vi "VernierTemp.vi"() -> ()   [LabVIEW 2019]
uses:
  <userlib>/MicroPython/VIs/uPythonX/uPythonX.xctl
panel:
  in  "Combined":T1(xcontrol)={"Port"="HighPeaksPYBD - ASRL114::INSTR", "All Code"="import micropython\nfrom bluetooth import BLE, UUID, FLAG_NOTIFY, FLAG_READ, FLAG_WRITE, FLAG_NOTIFY\nfrom micropython import const\nimport time\nimport struct\n\nmicropython.alloc_emergency_exception_buf(100)\n\nimport gc,utime\nimport pyb, micropython\nimport LPF2Class\n\n# Name, Format [# datasets, type, figures, decimals], raw [min,max], Percent, SI, Symbol,functionMap, view\nmode0 = ['LPF2-DETECT',[1,LPF2Class.DATA8,3,0],[0,10],[0,100],[0,10],'',[LPF2Class.ABSOLUTE,0],True]\nmode1 = ['LPF2-COUNT',[1,LPF2Class.DATA8,4,0],[0,100],[0,100],[0,100],'CNT',[LPF2Class.ABSOLUTE,0],True]\nmode2 = ['LPF2-CAL',[3,LPF2Class.DATA16,3,0],[0,1023],[0,100],[0,1023],'RAW',[LPF2Class.ABSOLUTE,0],False]\nmodes = [mode0,mode1,mode2]\n\nred_led=pyb.LED(1)\ngreen_led = pyb.LED(2)\nred_led.on()\n\nlpf2 = LPF2Class.LPF2(1, 'Y1', 'Y2', modes, 35, timer = 4, freq = 5)    # PyBoard\nlpf2.initialize()\n\nwhile True:\n     if not lpf2.connected:\n          lpf2.sendTimer.callback(None)\n          red_led.on()\n          utime.sleep_ms(200)\n          lpf2.initialize()\n     else:\n          red_led.off()\n          lpf2.current_mode = 0\n          lpf2.load_payload_char(4)\n          break\n\n#For debug, specify sensor to be found here:\nGDX_SENSOR_ORDER_CODE = \"GDX-TMP\" #Found on product label\nGDX_SENSOR_SN_LAST3 = \"4S7\"      #Last 3 digits of serial number found on product label\n\n# Bluetooth IRQ handler states. Commented out Subscriber conditions since this is for a central\n#_IRQ_CENTRAL_CONNECT                 = const(1 << 0)\n#_IRQ_CENTRAL_DISCONNECT              = const(1 << 1)\n#_IRQ_GATTS_WRITE                     = const(1 << 2)\n#_IRQ_GATTS_READ_REQUEST              = const(1 << 3)\n_IRQ_SCAN_RESULT                     = const(1 << 4)\n_IRQ_SCAN_COMPLETE                   = const(1 << 5)\n_IRQ_PERIPHERAL_CONNECT              = const(1 << 6)\n_IRQ_PERIPHERAL_DISCONNECT           = const(1 << 7)\n_IRQ_GATTC_SERVICE_RESULT            = const(1 << 8)\n_IRQ_GATTC_CHARACTERISTIC_RESULT     = const(1 << 9)\n_IRQ_GATTC_DESCRIPTOR_RESULT         = const(1 << 10)\n_IRQ_GATTC_READ_RESULT               = const(1 << 11)\n_IRQ_GATTC_WRITE_STATUS              = const(1 << 12)\n_IRQ_GATTC_NOTIFY                    = const(1 << 13)\n_IRQ_GATTC_INDICATE                  = const(1 << 14)\n\n#Go Direct specific UUIDs for D2PIO (our protocol) communication.\nSERVICE_UUID                        = \"d91714ef-28b9-4f91-ba16-f0d9a604f112\"\nCMD_CHARACTERISTIC_UUID             = \"f4bf14a6-c7d5-4b6d-8aa8-df1a7c83adcb\"\nRESPONSE_CHARACTERISTIC_UUID        = \"b41e6675-a329-40e0-aa01-44d2f444babe\"\n\n#Go Direct command and expected responses\nINIT                                = b'\\x58\\x19\\xfe\\x3f\\x1a\\xa5\\x4a\\x06\\x49\\x07\\x48\\x08\\x47\\x09\\x46\\x0a\\x45\\x0b\\x44\\x0c\\x43\\x0d\\x42\\x0e\\x41'\nINIT_RESPONSE                       = b'\\xb8\\x1a\\x00\\xe0\\x1a\\xfe\\x55\\xaa\\x56\\xa9\\x57\\xa8\\x58\\xa7\\x59\\xa6\\x5a\\xa5\\x5b\\xa4\\x5c\\xa3\\x5d\\xa2\\x5e\\xa1'\nGET_STATUS_CMD                      = b'\\x58\\x05\\xfd\\x6a\\x10'\n#GET_STATUS_RESPONSE                 = b'\\x98\\x12\\x01\\x0d\\x10\\xfd\\x00\\x00\\x04\\x01\\x00\\x00\\x04\\x01\\x00\\x00\\x4b\\x00' Example only. State/Sensor dependent\nAVAILABLE_CHANNELS_CMD              = b'\\x58\\x05\\xfc\\xaa\\x51'\n#AVAILABLE_CHANNELS_RESP             = b'\\x98\\x0a\\x01\\xf4\\x51\\xfe\\x02\\x00\\x00\\x00' Example only. State/Sensor dependent\n#sample period of 0.1 sec  = 01 86 a0\n#smaple period of 1.0 sec  = 0f 42 40\nSET_MEASUREMENT_PERIOD_CMD          = b'\\x58\\x0f\\xfb\\xa3\\x1b\\xff\\x00\\x40\\x42\\x0f\\x00\\x00\\x00\\x00\\x00'\n#SET_MEASUREMENT_PERIOD_RESP         = b'\\x98\\x10\\x03\\xe7\\x1b\\xfb \\xff\\x00\\xa0\\x86\\x01\\x00\\x00\\x00\\x00\\x00' Example only. State/Sensor dependent\nSTART_MEASUREMENTS_CMD              = b'\\x58\\x13\\xfa\\x7f\\x18\\xff\\x01\\x02\\x00\\x00\\x00\\x00\\x00\\x00\\x00\\x00\\x00\\x00\\x00'\n#START_MEASUREMENTS_CMD              = b'\\x58\\x13\\xfa\\x7f\\x18\\xff\\x00\\x02\\x00\\x00\\x00\\x00\\x00\\x00\\x00\\x00\\x00\\x00\\x00'\n#START_MEASUREMENTS_RESP             = b'\\x98\\x07\\x04\\xb5\\x18\\xfa\\x00' Example only. State/Sensor dependent\nSTOP_MEASUREMENTS_CMD               = b'\\x58\\x0b\\xf9\\x70\\x19\\xff\\x00\\xff\\xff\\xff\\xff'\nSTOP_MEASUREMENTS_RESP              = b'\\x98\\x07\\x05\\xb6\\x19\\xf9\\x00'\n\n\nglobal scanning_flag\nscanning_flag = False\n\nclass BLEPeripheral:\n  def __init__(self):\n    self._addr_type = None\n    self._addr = bytearray(5)\n    self._conn_handle = None\n    self._connect_status = False\n    self._rssi = None\n    self._name = None\n    #characteristic info from querry\n    self._cmdhandle = 20\n    self._resphandle = 22\n    self._command = bytearray()\n    self._response = bytearray()\n    #D2PIO Protocol\n    self._rolling_counter = None\n\n  def connected(self):\n   pass\n\n\ndef adv_decode(adv_type, data):\n    i = 0\n    while i + 1 < len(data):\n        if data[i + 1] == adv_type:\n            return data[i + 2:i + data[i] + 1]\n        i += 1 + data[i]\n    return None\n\ndef adv_decode_name(data):\n    n = adv_decode(0x09, data)\n    if n:\n        return n.decode('utf-8')\n    return data\n\ndef bt_irq(event, data):\n  global scanning_flag\n  if event == _IRQ_SCAN_RESULT:\n    # A single scan result.\n    addr_type, addr, connectable, rssi, adv_data = data\n    if adv_decode_name(adv_data).startswith(GDX_SENSOR_ORDER_CODE) and connectable:\n        if adv_decode_name(adv_data).endswith(GDX_SENSOR_SN_LAST3):\n            print(addr_type, addr, connectable, rssi, adv_decode_name(adv_data))\n            bledevice._addr[:] = addr\n            bledevice._addr_type = addr_type\n            bledevice._rssi = rssi\n        pass\n  elif event == _IRQ_SCAN_COMPLETE:\n    # Scan duration finished or manually stopped.\n    #print('scan complete')\n    scanning_flag = False\n    pass\n  elif event == _IRQ_PERIPHERAL_CONNECT:\n    # A successful gap_connect().\n    conn_handle, addr_type, addr = data\n    bledevice._conn_handle = conn_handle\n    print(\"Connected to \" + str(conn_handle) + str(addr_type))\n    scanning_flag = False\n  elif event == _IRQ_PERIPHERAL_DISCONNECT:\n    # A successful gap_connect().\n    conn_handle, addr_type, addr = data\n    print(\"Disconnected\")\n    scanning_flag = False\n  elif event == _IRQ_GATTC_SERVICE_RESULT:\n    # Called for each service found by gattc_discover_services().\n    conn_handle, start_handle, end_handle, uuid = data\n    print(\"Service\", conn_handle, start_handle, end_handle, uuid)\n    scanning_flag = False\n  elif event == _IRQ_GATTC_CHARACTERISTIC_RESULT:\n    # Called for each characteristic found by gattc_discover_services().\n    conn_handle, def_handle, value_handle, properties, uuid = data\n    print(\"Characteristic\", conn_handle, def_handle, value_handle, properties, uuid)\n    scanning_flag = False\n  elif event == _IRQ_GATTC_DESCRIPTOR_RESULT:\n    # Called for each characteristic found by gattc_discover_services().\n    conn_handle, dsc_handle, uuid = data\n    print(\"Descriptor\", conn_handle, dsc_handle, uuid)\n    scanning_flag = False\n  elif event == _IRQ_GATTC_READ_RESULT:\n    # A gattc_read() has completed.\n    conn_handle, value_handle, char_data = data\n    bledevice._response[:] = char_data            \n    print(conn_handle, value_handle, char_data)\n    scanning_flag = False\n  elif event == _IRQ_GATTC_WRITE_STATUS:\n    # A gattc_write() has completed.\n    conn_handle, value_handle, status = data\n    print(\"Data write\" , conn_handle, value_handle, status)\n    scanning_flag = False\n  elif event == _IRQ_GATTC_NOTIFY:\n    # A peripheral has sent a notify request.\n    conn_handle, value_handle, notify_data = data\n #   print(\"Notify\", value_handle, notify_data)\n #   if conn_handle == bledevice._conn_handle and value_handle == bledevice._resphandle:\n    bledevice._response[:] = notify_data\n    scanning_flag = False\n  else :\n    print(\"IRQ Number\", event)\n\n\ndef GDX_calculate_checksum(buff):\n    length = int(buff[1])\n    checksum = -1 * int(buff[3])\n\n    for i in range(0,length):\n        checksum += int(buff[i])\n        checksum = checksum & 0xFF\n\n        if checksum < 0 or checksum > 255:\n            return 0\n\n    return checksum\n\ndef GDX_SendInit(PassedBLEDevice):\n    # Reset the rolling packet counter\n    PassedBLEDevice._rolling_counter = 0xFF\n    PassedBLEDevice._command = INIT\n    # Populate the packet header bytes\n    workinglist = list(PassedBLEDevice._command)\n    workinglist[1] = len(PassedBLEDevice._command)\n    workinglist[2] = PassedBLEDevice._rolling_counter\n    PassedBLEDevice._rolling_counter = PassedBLEDevice._rolling_counter -1\n    workinglist[3] = 0 \n    workinglist[3] = GDX_calculate_checksum(workinglist)\n    PassedBLEDevice._command = bytearray(workinglist)\n    scanning_flag = True\n    bt.gattc_write(PassedBLEDevice._conn_handle, PassedBLEDevice._cmdhandle, PassedBLEDevice._command,True)\n    return\n\ndef GDX_GetStatus(PassedBLEDevice):\n    PassedBLEDevice._command = GET_STATUS_CMD\n    # Populate the packet header bytes\n    workinglist = list(PassedBLEDevice._command)\n    workinglist[1] = len(PassedBLEDevice._command)\n    workinglist[2] = PassedBLEDevice._rolling_counter\n    PassedBLEDevice._rolling_counter = PassedBLEDevice._rolling_counter -1\n    workinglist[3] = 0 \n    workinglist[3] = GDX_calculate_checksum(workinglist)\n    PassedBLEDevice._command = bytearray(workinglist)\n    print(\"GetStatus CMD\", PassedBLEDevice._command)\n    bt.gattc_write(PassedBLEDevice._conn_handle, PassedBLEDevice._cmdhandle, PassedBLEDevice._command,True)\n    return\n\ndef GDX_AvalCh(PassedBLEDevice):\n    PassedBLEDevice._command = AVAILABLE_CHANNELS_CMD\n    # Populate the packet header bytes\n    workinglist = list(PassedBLEDevice._command)\n    workinglist[1] = len(PassedBLEDevice._command)\n    workinglist[2] = PassedBLEDevice._rolling_counter\n    PassedBLEDevice._rolling_counter = PassedBLEDevice._rolling_counter -1\n    workinglist[3] = 0 \n    workinglist[3] = GDX_calculate_checksum(workinglist)\n    PassedBLEDevice._command = bytearray(workinglist)\n    print(\"Available Channels CMD\", PassedBLEDevice._command)\n    bt.gattc_write(PassedBLEDevice._conn_handle, PassedBLEDevice._cmdhandle, PassedBLEDevice._command,True)\n    return\n\ndef GDX_SetPeriod(PassedBLEDevice):\n    bt2 = BLE()\n    PassedBLEDevice._command = SET_MEASUREMENT_PERIOD_CMD\n    workinglist = list(PassedBLEDevice._command)\n    workinglist[1] = len(PassedBLEDevice._command)\n    workinglist[2] = PassedBLEDevice._rolling_counter\n    PassedBLEDevice._rolling_counter = PassedBLEDevice._rolling_counter -1\n    workinglist[3] = 0 \n    workinglist[3] = GDX_calculate_checksum(workinglist)\n    PassedBLEDevice._command = bytearray(workinglist)\n    print(\"Set Period\", PassedBLEDevice._command, PassedBLEDevice._conn_handle, PassedBLEDevice._cmdhandle)\n    bt2.gattc_write(PassedBLEDevice._conn_handle, PassedBLEDevice._cmdhandle, PassedBLEDevice._command,True)\n    return\n\ndef GDX_StartMeasurement(PassedBLEDevice):\n    bt2 = BLE()\n    PassedBLEDevice._command = START_MEASUREMENTS_CMD\n    workinglist = list(PassedBLEDevice._command)\n    workinglist[1] = len(PassedBLEDevice._command)\n    workinglist[2] = PassedBLEDevice._rolling_counter\n    PassedBLEDevice._rolling_counter = PassedBLEDevice._rolling_counter -1\n    workinglist[3] = 0 \n    workinglist[3] = GDX_calculate_checksum(workinglist)\n    PassedBLEDevice._command = bytearray(workinglist)\n    print(\"Start Measurements\", PassedBLEDevice._command, PassedBLEDevice._conn_handle, PassedBLEDevice._cmdhandle)\n    bt2.gattc_write(PassedBLEDevice._conn_handle, PassedBLEDevice._cmdhandle, PassedBLEDevice._command,True)\n    return\n\ndef GDX_StopMeasurement(PassedBLEDevice):\n    PassedBLEDevice._command = STOP_MEASUREMENTS_CMD\n    # Populate the packet header bytes\n    workinglist = list(PassedBLEDevice._command)\n    workinglist[1] = len(PassedBLEDevice._command)\n    workinglist[2] = PassedBLEDevice._rolling_counter\n    PassedBLEDevice._rolling_counter = PassedBLEDevice._rolling_counter -1\n    workinglist[3] = 0 \n    workinglist[3] = GDX_calculate_checksum(workinglist)\n    PassedBLEDevice._command = bytearray(workinglist)\n    bt.gattc_write(PassedBLEDevice._conn_handle, PassedBLEDevice._cmdhandle, PassedBLEDevice._command,True)\n    return\n\n'''\nTest program to take samples for 10 sec. at 1 sec. intervals\n'''\n#Scan for sensor \nbt = BLE()\nbledevice = BLEPeripheral()\nbt.irq(handler=bt_irq)\nbt.active(True)\nscanning_flag = True\nbt.gap_scan(2000, 1000, 1000)\nwhile scanning_flag:\n    pass\n\n#we have our sensor, now connect\nscanning_flag = True\nbt.gap_connect(bledevice._addr_type,bledevice._addr,)\nwhile scanning_flag:\n    pass\nprint('successful conn handle: ' + str(bledevice._conn_handle))\n\ntime.sleep_ms(500)\nbledevice._command = b'\\x01\\x00' #enable notification on characteristic\nbt.gattc_write(bledevice._conn_handle, 23, bledevice._command,False)\nwhile scanning_flag:\n    pass\nscanning_flag = True\nbt.gattc_read(bledevice._conn_handle,23)\n\nGDX_SendInit(bledevice)\n\nGDX_SetPeriod(bledevice)\n\nscanning_flag = True\nGDX_StartMeasurement(bledevice)\nwhile scanning_flag:        #wait for IRQ to clear flag\n    pass\n\nscanning_flag = True\nwhile scanning_flag:        #wait for IRQ to clear flag\n    pass\nprint(\"Start Measurements response\", bledevice._response)\n\nsamples = 0\nwhile samples < 10 :\n    scanning_flag = True\n    while scanning_flag:    #wait for IRQ to clear flag\n        pass\n    #time.sleep_ms(500)\n    samples = samples + 1\n    value = struct.unpack(\"<f\",bledevice._response[9:])[0]\n    print(\"Data sample number =\", bledevice._response[2] , struct.unpack(\"<f\",bledevice._response[9:]))\n    print(value, int(value))\nscanning_flag = True\nwhile scanning_flag:        #wait for IRQ to clear flag\n    pass\nprint(\"Measurements Stopped\")\n\n\n"}
  in  "Spike":T2(xcontrol)={"VISA Refnum in"="Spike - ASRL102::INSTR", "Python Code"="import hub,utime\n\nhub.port.B.info()\n\n# if info comes back with None - then you have to restart the pybaord\ni=0\n\nwhile True:\n     try:\n          value = hub.port.B.device.get()[0]\n          #print(value)\n          hub.display.show(str(value))\n          utime.sleep(0.1)\n     except:\n          utime.sleep(1)\n     \n"}
  in  "PYBD":T2(xcontrol)={"VISA Refnum in"="HighPeaksPYBD - ASRL114::INSTR", "Python Code"="import gc,utime\nimport pyb, micropython\nimport LPF2Class\n\nmicropython.alloc_emergency_exception_buf(200)\n\n# Name, Format [# datasets, type, figures, decimals], raw [min,max], Percent, SI, Symbol,functionMap, view\nmode0 = ['LPF2-DETECT',[1,LPF2Class.DATA8,3,0],[0,10],[0,100],[0,10],'',[LPF2Class.ABSOLUTE,0],True]\nmode1 = ['LPF2-COUNT',[1,LPF2Class.DATA8,4,0],[0,100],[0,100],[0,100],'CNT',[LPF2Class.ABSOLUTE,0],True]\nmode2 = ['LPF2-CAL',[3,LPF2Class.DATA16,3,0],[0,1023],[0,100],[0,1023],'RAW',[LPF2Class.ABSOLUTE,0],False]\nmodes = [mode0,mode1,mode2]\n\nred_led=pyb.LED(1)\ngreen_led = pyb.LED(2)\nred_led.on()\n\nlpf2 = LPF2Class.LPF2(1, 'Y1', 'Y2', modes, 35, timer = 4, freq = 5)    # PyBoard\nlpf2.initialize()\n\nvalue = 0\n\n# Loop\nwhile True:\n     if not lpf2.connected:\n          lpf2.sendTimer.callback(None)\n          red_led.on()\n          utime.sleep_ms(200)\n          lpf2.initialize()\n     else:\n          red_led.off()\n          \n          lpf2.current_mode = 0\n#          lpf2.load_payload_charArray(bytes([1,2,3,4]))\n#          lpf2.current_mode = 1\n          lpf2.load_payload_char(value)\n          \n          value = value + 1 if value <9 else 0\n          data = lpf2.readIt(timeout = 0.01)\n\n          utime.sleep_ms(90)\n"}
  in  "uPythonX":T1(xcontrol)={"Port"="HighPeaksPYBD - ASRL114::INSTR", "All Code"="import micropython\nfrom bluetooth import BLE, UUID, FLAG_NOTIFY, FLAG_READ, FLAG_WRITE, FLAG_NOTIFY\nfrom micropython import const\nimport time\nimport struct\n\nmicropython.alloc_emergency_exception_buf(100)\n\n#For debug, specify sensor to be found here:\nGDX_SENSOR_ORDER_CODE = \"GDX-TMP\" #Found on product label\nGDX_SENSOR_SN_LAST3 = \"4S7\"      #Last 3 digits of serial number found on product label\n\n# Bluetooth IRQ handler states. Commented out Subscriber conditions since this is for a central\n#_IRQ_CENTRAL_CONNECT                 = const(1 << 0)\n#_IRQ_CENTRAL_DISCONNECT              = const(1 << 1)\n#_IRQ_GATTS_WRITE                     = const(1 << 2)\n#_IRQ_GATTS_READ_REQUEST              = const(1 << 3)\n_IRQ_SCAN_RESULT                     = const(1 << 4)\n_IRQ_SCAN_COMPLETE                   = const(1 << 5)\n_IRQ_PERIPHERAL_CONNECT              = const(1 << 6)\n_IRQ_PERIPHERAL_DISCONNECT           = const(1 << 7)\n_IRQ_GATTC_SERVICE_RESULT            = const(1 << 8)\n_IRQ_GATTC_CHARACTERISTIC_RESULT     = const(1 << 9)\n_IRQ_GATTC_DESCRIPTOR_RESULT         = const(1 << 10)\n_IRQ_GATTC_READ_RESULT               = const(1 << 11)\n_IRQ_GATTC_WRITE_STATUS              = const(1 << 12)\n_IRQ_GATTC_NOTIFY                    = const(1 << 13)\n_IRQ_GATTC_INDICATE                  = const(1 << 14)\n\n#Go Direct specific UUIDs for D2PIO (our protocol) communication.\nSERVICE_UUID                        = \"d91714ef-28b9-4f91-ba16-f0d9a604f112\"\nCMD_CHARACTERISTIC_UUID             = \"f4bf14a6-c7d5-4b6d-8aa8-df1a7c83adcb\"\nRESPONSE_CHARACTERISTIC_UUID        = \"b41e6675-a329-40e0-aa01-44d2f444babe\"\n\n#Go Direct command and expected responses\nINIT                                = b'\\x58\\x19\\xfe\\x3f\\x1a\\xa5\\x4a\\x06\\x49\\x07\\x48\\x08\\x47\\x09\\x46\\x0a\\x45\\x0b\\x44\\x0c\\x43\\x0d\\x42\\x0e\\x41'\nINIT_RESPONSE                       = b'\\xb8\\x1a\\x00\\xe0\\x1a\\xfe\\x55\\xaa\\x56\\xa9\\x57\\xa8\\x58\\xa7\\x59\\xa6\\x5a\\xa5\\x5b\\xa4\\x5c\\xa3\\x5d\\xa2\\x5e\\xa1'\nGET_STATUS_CMD                      = b'\\x58\\x05\\xfd\\x6a\\x10'\n#GET_STATUS_RESPONSE                 = b'\\x98\\x12\\x01\\x0d\\x10\\xfd\\x00\\x00\\x04\\x01\\x00\\x00\\x04\\x01\\x00\\x00\\x4b\\x00' Example only. State/Sensor dependent\nAVAILABLE_CHANNELS_CMD              = b'\\x58\\x05\\xfc\\xaa\\x51'\n#AVAILABLE_CHANNELS_RESP             = b'\\x98\\x0a\\x01\\xf4\\x51\\xfe\\x02\\x00\\x00\\x00' Example only. State/Sensor dependent\n#sample period of 0.1 sec  = 01 86 a0\n#smaple period of 1.0 sec  = 0f 42 40\nSET_MEASUREMENT_PERIOD_CMD          = b'\\x58\\x0f\\xfb\\xa3\\x1b\\xff\\x00\\x40\\x42\\x0f\\x00\\x00\\x00\\x00\\x00'\n#SET_MEASUREMENT_PERIOD_RESP         = b'\\x98\\x10\\x03\\xe7\\x1b\\xfb \\xff\\x00\\xa0\\x86\\x01\\x00\\x00\\x00\\x00\\x00' Example only. State/Sensor dependent\nSTART_MEASUREMENTS_CMD              = b'\\x58\\x13\\xfa\\x7f\\x18\\xff\\x01\\x02\\x00\\x00\\x00\\x00\\x00\\x00\\x00\\x00\\x00\\x00\\x00'\n#START_MEASUREMENTS_CMD              = b'\\x58\\x13\\xfa\\x7f\\x18\\xff\\x00\\x02\\x00\\x00\\x00\\x00\\x00\\x00\\x00\\x00\\x00\\x00\\x00'\n#START_MEASUREMENTS_RESP             = b'\\x98\\x07\\x04\\xb5\\x18\\xfa\\x00' Example only. State/Sensor dependent\nSTOP_MEASUREMENTS_CMD               = b'\\x58\\x0b\\xf9\\x70\\x19\\xff\\x00\\xff\\xff\\xff\\xff'\nSTOP_MEASUREMENTS_RESP              = b'\\x98\\x07\\x05\\xb6\\x19\\xf9\\x00'\n\n\nglobal scanning_flag\nscanning_flag = False\n\nclass BLEPeripheral:\n  def __init__(self):\n    self._addr_type = None\n    self._addr = bytearray(5)\n    self._conn_handle = None\n    self._connect_status = False\n    self._rssi = None\n    self._name = None\n    #characteristic info from querry\n    self._cmdhandle = 20\n    self._resphandle = 22\n    self._command = bytearray()\n    self._response = bytearray()\n    #D2PIO Protocol\n    self._rolling_counter = None\n\n  def connected(self):\n   pass\n\n\ndef adv_decode(adv_type, data):\n    i = 0\n    while i + 1 < len(data):\n        if data[i + 1] == adv_type:\n            return data[i + 2:i + data[i] + 1]\n        i += 1 + data[i]\n    return None\n\ndef adv_decode_name(data):\n    n = adv_decode(0x09, data)\n    if n:\n        return n.decode('utf-8')\n    return data\n\ndef bt_irq(event, data):\n  global scanning_flag\n  if event == _IRQ_SCAN_RESULT:\n    # A single scan result.\n    addr_type, addr, connectable, rssi, adv_data = data\n    if adv_decode_name(adv_data).startswith(GDX_SENSOR_ORDER_CODE) and connectable:\n        if adv_decode_name(adv_data).endswith(GDX_SENSOR_SN_LAST3):\n            print(addr_type, addr, connectable, rssi, adv_decode_name(adv_data))\n            bledevice._addr[:] = addr\n            bledevice._addr_type = addr_type\n            bledevice._rssi = rssi\n        pass\n  elif event == _IRQ_SCAN_COMPLETE:\n    # Scan duration finished or manually stopped.\n    #print('scan complete')\n    scanning_flag = False\n    pass\n  elif event == _IRQ_PERIPHERAL_CONNECT:\n    # A successful gap_connect().\n    conn_handle, addr_type, addr = data\n    bledevice._conn_handle = conn_handle\n    print(\"Connected to \" + str(conn_handle) + str(addr_type))\n    scanning_flag = False\n  elif event == _IRQ_PERIPHERAL_DISCONNECT:\n    # A successful gap_connect().\n    conn_handle, addr_type, addr = data\n    print(\"Disconnected\")\n    scanning_flag = False\n  elif event == _IRQ_GATTC_SERVICE_RESULT:\n    # Called for each service found by gattc_discover_services().\n    conn_handle, start_handle, end_handle, uuid = data\n    print(\"Service\", conn_handle, start_handle, end_handle, uuid)\n    scanning_flag = False\n  elif event == _IRQ_GATTC_CHARACTERISTIC_RESULT:\n    # Called for each characteristic found by gattc_discover_services().\n    conn_handle, def_handle, value_handle, properties, uuid = data\n    print(\"Characteristic\", conn_handle, def_handle, value_handle, properties, uuid)\n    scanning_flag = False\n  elif event == _IRQ_GATTC_DESCRIPTOR_RESULT:\n    # Called for each characteristic found by gattc_discover_services().\n    conn_handle, dsc_handle, uuid = data\n    print(\"Descriptor\", conn_handle, dsc_handle, uuid)\n    scanning_flag = False\n  elif event == _IRQ_GATTC_READ_RESULT:\n    # A gattc_read() has completed.\n    conn_handle, value_handle, char_data = data\n    bledevice._response[:] = char_data            \n    print(conn_handle, value_handle, char_data)\n    scanning_flag = False\n  elif event == _IRQ_GATTC_WRITE_STATUS:\n    # A gattc_write() has completed.\n    conn_handle, value_handle, status = data\n    print(\"Data write\" , conn_handle, value_handle, status)\n    scanning_flag = False\n  elif event == _IRQ_GATTC_NOTIFY:\n    # A peripheral has sent a notify request.\n    conn_handle, value_handle, notify_data = data\n #   print(\"Notify\", value_handle, notify_data)\n #   if conn_handle == bledevice._conn_handle and value_handle == bledevice._resphandle:\n    bledevice._response[:] = notify_data\n    scanning_flag = False\n  else :\n    print(\"IRQ Number\", event)\n\n\ndef GDX_calculate_checksum(buff):\n    length = int(buff[1])\n    checksum = -1 * int(buff[3])\n\n    for i in range(0,length):\n        checksum += int(buff[i])\n        checksum = checksum & 0xFF\n\n        if checksum < 0 or checksum > 255:\n            return 0\n\n    return checksum\n\ndef GDX_SendInit(PassedBLEDevice):\n    # Reset the rolling packet counter\n    PassedBLEDevice._rolling_counter = 0xFF\n    PassedBLEDevice._command = INIT\n    # Populate the packet header bytes\n    workinglist = list(PassedBLEDevice._command)\n    workinglist[1] = len(PassedBLEDevice._command)\n    workinglist[2] = PassedBLEDevice._rolling_counter\n    PassedBLEDevice._rolling_counter = PassedBLEDevice._rolling_counter -1\n    workinglist[3] = 0 \n    workinglist[3] = GDX_calculate_checksum(workinglist)\n    PassedBLEDevice._command = bytearray(workinglist)\n    scanning_flag = True\n    bt.gattc_write(PassedBLEDevice._conn_handle, PassedBLEDevice._cmdhandle, PassedBLEDevice._command,True)\n    return\n\ndef GDX_GetStatus(PassedBLEDevice):\n    PassedBLEDevice._command = GET_STATUS_CMD\n    # Populate the packet header bytes\n    workinglist = list(PassedBLEDevice._command)\n    workinglist[1] = len(PassedBLEDevice._command)\n    workinglist[2] = PassedBLEDevice._rolling_counter\n    PassedBLEDevice._rolling_counter = PassedBLEDevice._rolling_counter -1\n    workinglist[3] = 0 \n    workinglist[3] = GDX_calculate_checksum(workinglist)\n    PassedBLEDevice._command = bytearray(workinglist)\n    print(\"GetStatus CMD\", PassedBLEDevice._command)\n    bt.gattc_write(PassedBLEDevice._conn_handle, PassedBLEDevice._cmdhandle, PassedBLEDevice._command,True)\n    return\n\ndef GDX_AvalCh(PassedBLEDevice):\n    PassedBLEDevice._command = AVAILABLE_CHANNELS_CMD\n    # Populate the packet header bytes\n    workinglist = list(PassedBLEDevice._command)\n    workinglist[1] = len(PassedBLEDevice._command)\n    workinglist[2] = PassedBLEDevice._rolling_counter\n    PassedBLEDevice._rolling_counter = PassedBLEDevice._rolling_counter -1\n    workinglist[3] = 0 \n    workinglist[3] = GDX_calculate_checksum(workinglist)\n    PassedBLEDevice._command = bytearray(workinglist)\n    print(\"Available Channels CMD\", PassedBLEDevice._command)\n    bt.gattc_write(PassedBLEDevice._conn_handle, PassedBLEDevice._cmdhandle, PassedBLEDevice._command,True)\n    return\n\ndef GDX_SetPeriod(PassedBLEDevice):\n    bt2 = BLE()\n    PassedBLEDevice._command = SET_MEASUREMENT_PERIOD_CMD\n    workinglist = list(PassedBLEDevice._command)\n    workinglist[1] = len(PassedBLEDevice._command)\n    workinglist[2] = PassedBLEDevice._rolling_counter\n    PassedBLEDevice._rolling_counter = PassedBLEDevice._rolling_counter -1\n    workinglist[3] = 0 \n    workinglist[3] = GDX_calculate_checksum(workinglist)\n    PassedBLEDevice._command = bytearray(workinglist)\n    print(\"Set Period\", PassedBLEDevice._command, PassedBLEDevice._conn_handle, PassedBLEDevice._cmdhandle)\n    bt2.gattc_write(PassedBLEDevice._conn_handle, PassedBLEDevice._cmdhandle, PassedBLEDevice._command,True)\n    return\n\ndef GDX_StartMeasurement(PassedBLEDevice):\n    bt2 = BLE()\n    PassedBLEDevice._command = START_MEASUREMENTS_CMD\n    workinglist = list(PassedBLEDevice._command)\n    workinglist[1] = len(PassedBLEDevice._command)\n    workinglist[2] = PassedBLEDevice._rolling_counter\n    PassedBLEDevice._rolling_counter = PassedBLEDevice._rolling_counter -1\n    workinglist[3] = 0 \n    workinglist[3] = GDX_calculate_checksum(workinglist)\n    PassedBLEDevice._command = bytearray(workinglist)\n    print(\"Start Measurements\", PassedBLEDevice._command, PassedBLEDevice._conn_handle, PassedBLEDevice._cmdhandle)\n    bt2.gattc_write(PassedBLEDevice._conn_handle, PassedBLEDevice._cmdhandle, PassedBLEDevice._command,True)\n    return\n\ndef GDX_StopMeasurement(PassedBLEDevice):\n    PassedBLEDevice._command = STOP_MEASUREMENTS_CMD\n    # Populate the packet header bytes\n    workinglist = list(PassedBLEDevice._command)\n    workinglist[1] = len(PassedBLEDevice._command)\n    workinglist[2] = PassedBLEDevice._rolling_counter\n    PassedBLEDevice._rolling_counter = PassedBLEDevice._rolling_counter -1\n    workinglist[3] = 0 \n    workinglist[3] = GDX_calculate_checksum(workinglist)\n    PassedBLEDevice._command = bytearray(workinglist)\n    bt.gattc_write(PassedBLEDevice._conn_handle, PassedBLEDevice._cmdhandle, PassedBLEDevice._command,True)\n    return\n\n'''\nTest program to take samples for 10 sec. at 1 sec. intervals\n'''\n#Scan for sensor \nbt = BLE()\nbledevice = BLEPeripheral()\nbt.irq(handler=bt_irq)\nbt.active(True)\nscanning_flag = True\nbt.gap_scan(2000, 1000, 1000)\nwhile scanning_flag:\n    pass\n\n#we have our sensor, now connect\nscanning_flag = True\nbt.gap_connect(bledevice._addr_type,bledevice._addr,)\nwhile scanning_flag:\n    pass\nprint('successful conn handle: ' + str(bledevice._conn_handle))\n\ntime.sleep_ms(500)\nbledevice._command = b'\\x01\\x00' #enable notification on characteristic\nbt.gattc_write(bledevice._conn_handle, 23, bledevice._command,False)\nwhile scanning_flag:\n    pass\nscanning_flag = True\nbt.gattc_read(bledevice._conn_handle,23)\n\nGDX_SendInit(bledevice)\n\nGDX_SetPeriod(bledevice)\n\nscanning_flag = True\nGDX_StartMeasurement(bledevice)\nwhile scanning_flag:        #wait for IRQ to clear flag\n    pass\n\nscanning_flag = True\nwhile scanning_flag:        #wait for IRQ to clear flag\n    pass\nprint(\"Start Measurements response\", bledevice._response)\n\nsamples = 0\nwhile samples < 10 :\n    scanning_flag = True\n    while scanning_flag:    #wait for IRQ to clear flag\n        pass\n    #time.sleep_ms(500)\n    samples = samples + 1\n    print(\"Data sample number =\", bledevice._response[2] , struct.unpack(\"<f\",bledevice._response[9:]))\n\nscanning_flag = True\nwhile scanning_flag:        #wait for IRQ to clear flag\n    pass\nprint(\"Measurements Stopped\")\n\n\n"}
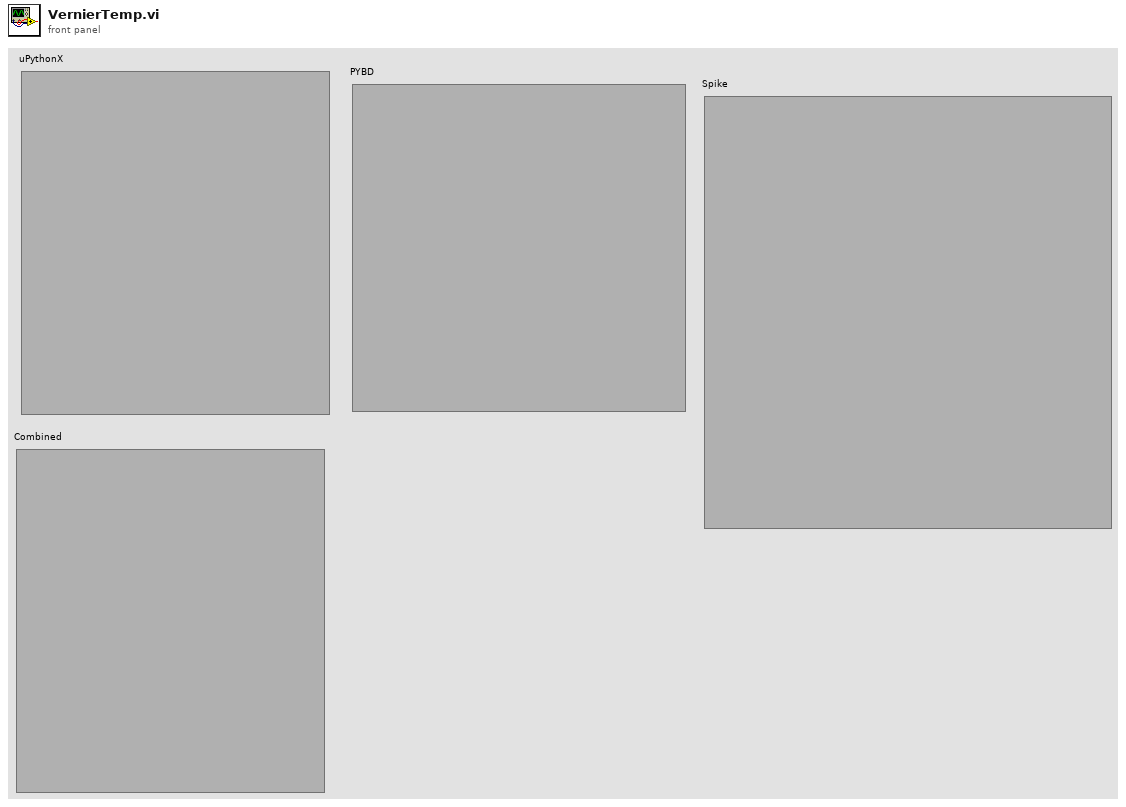
[diagram p1: front panel]
types:
  T1 = cluster{"Port":refnum<visa-resource-name>, "All Code":string}
  T2 = cluster{"VISA Refnum in":refnum<visa-resource-name>, "Python Code":string}
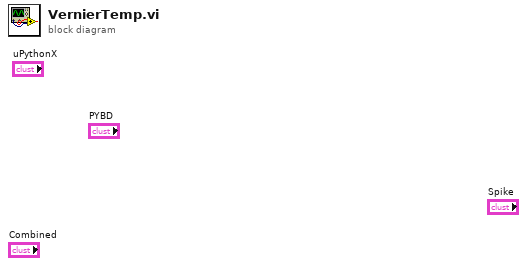
[diagram p0: block diagram]
diagram:
